vi "DLL Retcode to VI Errcode.vi"(7 "Driver VI No":T1, 8 "error in (no error)":errorcluster, 11 "DLL Return Code":i32 format="%x") -> (0 "error out":errorcluster, 3 "VI Error Code":i32)   [LabVIEW 2014, in "Keyence LJ-V7000.lvlib"]
uses:
  Keyence LJ-V7000.lvlib
  Public/constant/Driver VI No.ctl
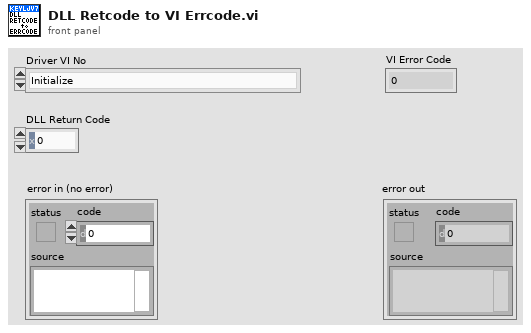
[diagram p1: front panel]
types:
  T1 = typedef "Keyence LJ-V7000.lvlib/Driver VI No.ctl" = enum16{"Initialize", "Close", "Reboot Controller", "Return to Factory State", "Get System Error", "Clear System Error", "Trigger", "Start Batch Measurements", "Stop Batch Measurements", "Auto Zero", "Timing", "Reset", "Clear Memory", "Set Setting", "Get Setting", "Initialize Setting", "Reflect Setting", "Update Write Settings Area", "Check Status of Saving to Save Area", "Set Time", "Get Time", "Change Program", "Read Active Program Number", "Read Measurement Data", "Read Profiles(for High-Speed Mode)", "Read Batch Profiles(for High-Speed Mode)", "Read Profiles(for Advanced Mode)", "Read Batch Profiles(for Advanced Mode)", "Start Storage", "Stop Storage", "Read Storage Status", "Read Data Storage Data", "Read Profile Storage Data", "Read Batch Profile Storage Data", "Start High-Speed Data Communication", "Stop High-Speed Data Communication", "Read Profiles(for High-Speed Communication)"}
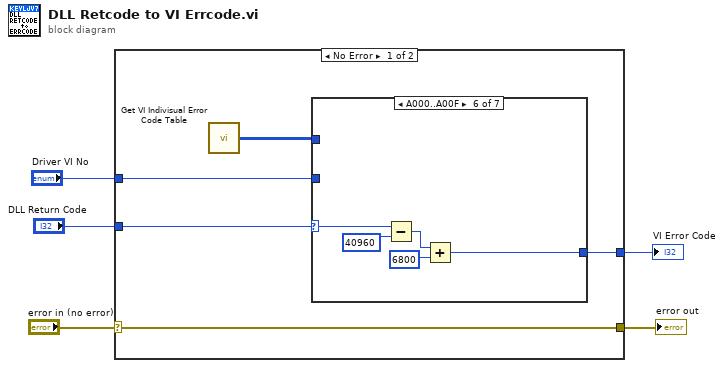
[diagram p0: block diagram]
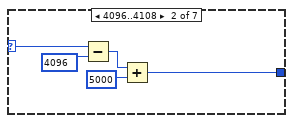
[diagram p3: hidden frame]
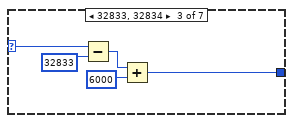
[diagram p4: hidden frame]
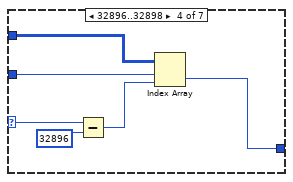
[diagram p5: hidden frame]
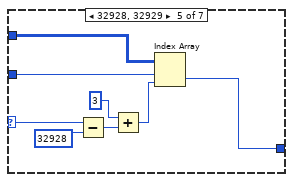
[diagram p6: hidden frame]
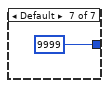
[diagram p7: hidden frame]
diagram:
  n1 = case shown="No Error" "error in (no error)" {
    selector: "error in (no error)" -> [w7 w42]
    tunnel: "DLL Return Code" -> [w10 w43]
    tunnel: "Driver VI No" -> [w9 _]
    tunnel: [w8 w43] -> w3
    tunnel: [w7 w42] -> w1
    frame No Error {
      n2 = call "Get VI Indivisual Error Code Table.vi"() -> ("Driver VI Individual Error Code Table"=w6:u16[][])  [unwired: 5 in]
      n3 = case shown="A000..A00F" w10 {
        selector: w10 -> [w11 w13 w18 w26 w34 w37 _]
        tunnel: [w11 w12 w17 w23 w32 w36 9999 ("l")] -> w8
        tunnel: w9 -> [_ _ _ w25 w33 _ _]
        tunnel: w6 -> [_ _ _ w22 w31 _ _]
        frame 0 {
        }
        frame 4096..4108 {
          n4 = Subtract(x=w13, y=4096) -> (x-y=w15:i32)
          n5 = Add(x=w15, y=5000) -> (x+y=w12:i32)
        }
        frame 32833, 32834 {
          n6 = Subtract(x=w18, y=32833) -> (x-y=w20:i32)
          n7 = Add(x=w20, y=6000) -> (x+y=w17:i32)
        }
        frame 32896..32898 {
          n8 = Subtract(x=w26, y=32896) -> (x-y=w24:i32)
          n9 = Index Array(array=w22, index (row)=w25, index (col)=w24) -> (element=w23:u16)
        }
        frame 32928, 32929 {
          n10 = Subtract(x=w34, y=32928) -> (x-y=w29:i32)
          n11 = Add(x=3, y=w29) -> (x+y=w28:i32)
          n12 = Index Array(array=w31, index (row)=w33, index (col)=w28) -> (element=w32:u16)
        }
        frame 40960..40975 {
          n13 = Subtract(x=w37, y=40960) -> (x-y=w39:i32)
          n14 = Add(x=w39, y=6800) -> (x+y=w36:i32)
        }
        frame Default {
        }
      }
    }
    frame Error {
    }
  }
  "VI Error Code" <- w3
  "error out" <- w1
